vi "Parameter Builder.vi"(8 "error in (no error)":errorcluster, 11 "Parameter Names":string[](array[string])) -> (0 "error out":errorcluster, 3 "Parameters":refnum<class "Parameter.lvclass">[](array[class]))   [LabVIEW 2023, in "HAF.lvlib" / "Parameter.lvclass"]
doc: "Given an array of names, returns an array of Parameters with the given name."
uses:
  Parameter.lvclass
  Parameter.lvclass/Parameter.ctl
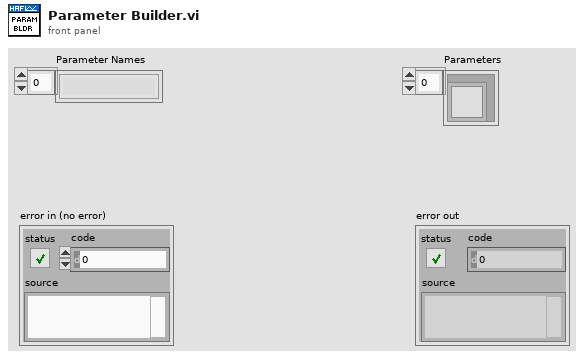
[diagram p1: front panel]
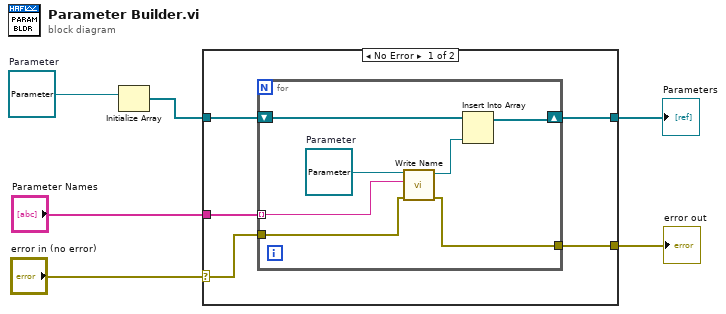
[diagram p0: block diagram]
diagram:
  w4 = refnum<class "Parameter.lvclass"> refnum  # Parameter
  n1 = Initialize Array(w4) -> (w3:refnum<class "Parameter.lvclass">[])  [unwired: 1 in]
  n2 = case shown="No Error" "error in (no error)" {
    selector: "error in (no error)" -> [w9 w20]
    tunnel: "Parameter Names" -> [w10 _]
    tunnel: w3 -> [w11 w19]
    tunnel: [w8 w20] -> w2
    tunnel: [w7 w19] -> w1
    frame No Error {
      n3 = for {
        shift-right: [w13] -> w7
        shift-left: w11 -> [w18]
        tunnel: w10 -> [w14] mode=indexing
        tunnel: w9 -> [w15]
        tunnel: [w12] -> w8
        w17 = refnum<class "Parameter.lvclass"> refnum  # Parameter
        n4 = call-dynamic "Write Name.vi"("error in (no error)"=w15, "Name"=w14, "Parameter in"=w17) -> ("error out"=w12:errorcluster, "Parameter out"=w16:refnum<class "Parameter.lvclass">)  [unwired: 7 in]
        n5 = Insert Into Array(array=w18, new element=w16) -> (w13:refnum<class "Parameter.lvclass">[])  [unwired: 1 in]
      }
    }
    frame Error {
    }
  }
  "Parameters" <- w1
  "error out" <- w2
